vi "Robot to Dashboard Comm.vi"   [LabVIEW 2012]
uses:
  Robot Global Data.vi
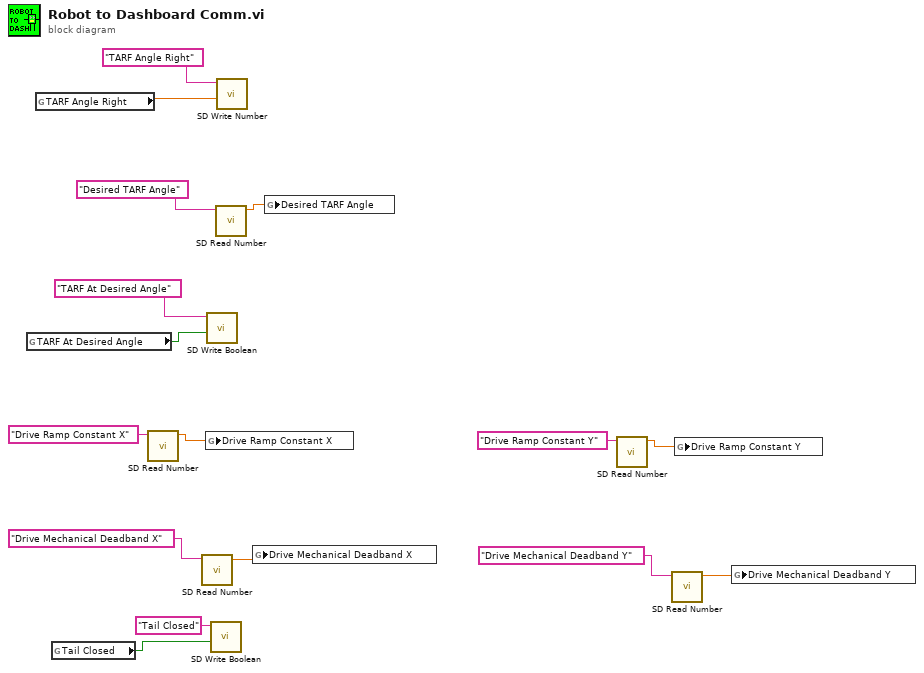
[diagram p0: block diagram]
diagram:
  n1 = global read "Robot Global Data.vi" "TARF At Desired Angle"() -> (w11:bool)
  n2 = global read "Robot Global Data.vi" "TARF Angle Right"() -> (w16:dbl)
  n3 = global read "Robot Global Data.vi" "Tail Closed"() -> (w1:bool)
  n4 = call <vilib>:"SD Read Number.vi"("Name"="Drive Ramp Constant X") -> ("Numeric"=w9:dbl)  [unwired: 8 in, 2 out]
  n5 = call <vilib>:"SD Read Number.vi"("Name"="Drive Mechanical Deadband X") -> ("Numeric"=w8:dbl)  [unwired: 8 in, 2 out]
  n6 = global write "Robot Global Data.vi" "Drive Ramp Constant X"(w9) -> ()
  n7 = call <vilib>:"SD Write Boolean.vi"("Boolean"=w11, "Name"="TARF At Desired Angle") -> ()  [unwired: 8 in, 2 out]
  n8 = call <vilib>:"SD Write Boolean.vi"("Boolean"=w1, "Name"="Tail Closed") -> ()  [unwired: 8 in, 2 out]
  n9 = call <vilib>:"SD Read Number.vi"("Name"="Desired TARF Angle") -> ("Numeric"=w12:dbl)  [unwired: 8 in, 2 out]
  n10 = call <vilib>:"SD Write Number.vi"("Numeric"=w16, "Name"="TARF Angle Right") -> ()  [unwired: 8 in, 2 out]
  n11 = global write "Robot Global Data.vi" "Drive Mechanical Deadband X"(w8) -> ()
  n12 = global write "Robot Global Data.vi" "Desired TARF Angle"(w12) -> ()
  n13 = call <vilib>:"SD Read Number.vi"("Name"="Drive Ramp Constant Y") -> ("Numeric"=w5:dbl)  [unwired: 8 in, 2 out]
  n14 = call <vilib>:"SD Read Number.vi"("Name"="Drive Mechanical Deadband Y") -> ("Numeric"=w4:dbl)  [unwired: 8 in, 2 out]
  n15 = global write "Robot Global Data.vi" "Drive Ramp Constant Y"(w5) -> ()
  n16 = global write "Robot Global Data.vi" "Drive Mechanical Deadband Y"(w4) -> ()
